vi "主.vi"() -> ()   [LabVIEW 2018]
uses:
  <vilib>/addons/database/Connection.llb/DB Tools Open Connec (String).vi
  <vilib>/addons/database/NI_Database_API.lvlib
  <vilib>/addons/database/Auxilliary.llb/DB Tools DataTypes.ctl
  <vilib>/addons/database/Auxilliary.llb/DB Tools Column Info.ctl
panel:
  out "密码":string[](array[string])
  out "账户":string[](array[string])
  in  "登录":bool
  in  "退出":bool
  in  "密码":string
  in  "用户":string
  in  "数据库路径":path
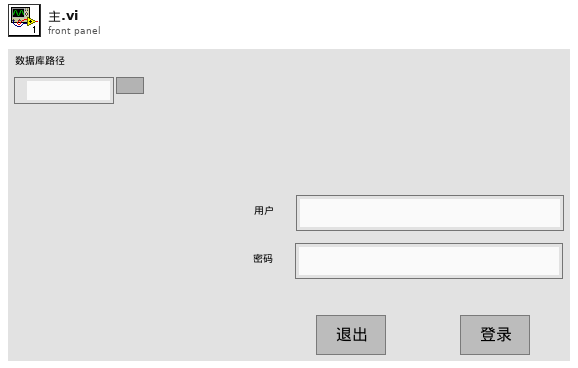
[diagram p1: front panel]
types:
  T1 = typedef "NI_Database_API.lvlib/DB Tools Column Info.ctl" = cluster{"column name":string, "data type":T2, "size":i32, "allow null?":bool}
  T2 = typedef "NI_Database_API.lvlib/DB Tools DataTypes.ctl" = enum16{"String", "Long (I32)", "Single (SGL)", "Double (DBL)", "Date/Time", "Binary"}
  T3 = typedef "NI_Database_API.lvlib/Conn ObjectReference.ctl" = refnum<k1>
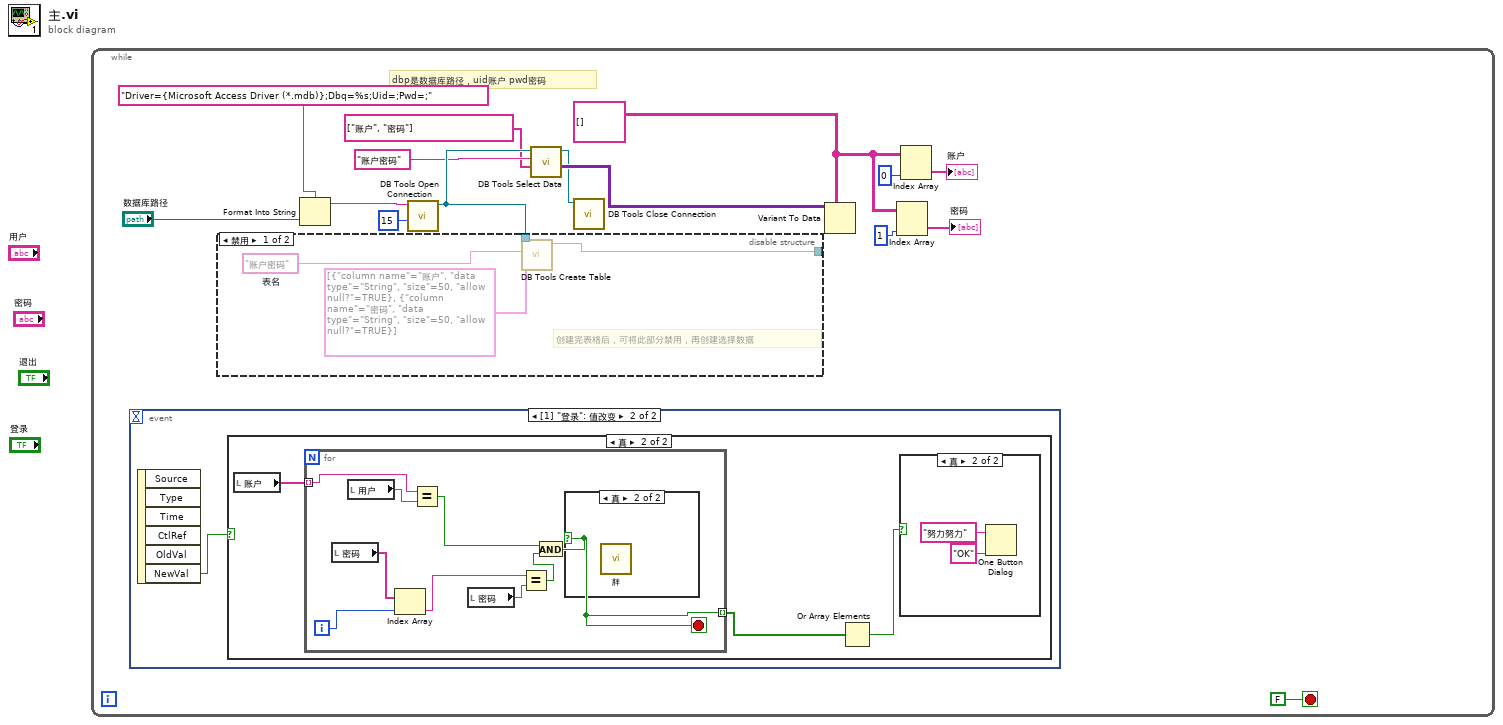
[diagram p0: block diagram]
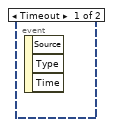
[diagram p3: hidden frame]
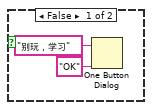
[diagram p6: hidden frame]
diagram:
  n1 = while {
    stop <- FALSE stop-if-true
    w7 = string[][] []
    # "dbp是数据库路径，uid账户 pwd密码"
    n2 = event shown="[1] \"登录\": 值改变" {
      selector: _ -> [_ _]
      dyn-events: _ -> [_ _]
      timeout: _ -> [_ _]
      event Timeout {
        n3 = event-data() -> ()  [unwired: 1 in, 3 out]
      }
      event "登录": Value Change {
        n4 = event-data() -> ("NewVal"=w20:bool)  [unwired: 1 in, 5 out]
        n5 = case shown="真" w20 {
          frame False {
          }
          frame True {
            n6 = local read "账户"() -> (w23:string[])
            n7 = for {
              tunnel: w23 -> [w34] mode=indexing
              tunnel: [w26] -> w21 mode=indexing
              i -> [w32]
              stop <- w26 stop-if-true
              n8 = local read "密码"() -> (w31:string[])
              n9 = local read "用户"() -> (w33:string)
              n10 = Index Array(array=w31, index=w32) -> (element=w30:string)
              n11 = Equal?(x=w34, y=w33) -> (x = y?=w28:bool)
              n12 = local read "密码"() -> (w29:string)
              n13 = Equal?(x=w30, y=w29) -> (x = y?=w27:bool)
              n14 = And(x=w28, y=w27) -> (x .and. y?=w26:bool)
              n15 = case shown="真" w26 {
                frame False {
                  n16 = One Button Dialog(message="别玩，学习" ("消息"), button name ("OK")="OK" ("按钮名称（“确定”）")) -> ()  [unwired: 1 out]
                }
                frame True {
                  n17 = call "胖.vi"() -> ()  [unwired: 12 in]
                }
              }
            }
            n18 = Or Array Elements(Boolean array=w21) -> (logical OR=w22:bool)
            n19 = case shown="真" w22 {
              frame False {
              }
              frame True {
                n20 = One Button Dialog(message="努力努力" ("消息"), button name ("OK")="OK" ("按钮名称（“确定”）")) -> ()  [unwired: 1 out]
              }
            }
          }
        }
      }
    }
    n21 = Format Into String(format string="Driver={Microsoft Access Driver (*.mdb)};Dbq=%s;Uid=;Pwd=;", "数据库路径") -> (resulting string=w13:string)  [unwired: 2 in, 1 out]
    n22 = call-poly <vilib>:"DB Tools Open Connection.vi"("connection timeout (15)"=15, "connection information"=w13) -> ("connection reference"=w11:T3)  [unwired: 6 in, 1 out]
    n23 = disable-structure shown="禁用" {
      disable-tunnel: [w19 _] -> _
      disable-tunnel: w11 -> [w16 _]
      frame Disabled {
        w18 = "账户密码"  # 表名
        # "创建完表格后，可将此部分禁用，再创建选择数据"
        n24 = call <vilib>:"DB Tools Create Table.vi"("column information"=T1[] [{"column name"="账户", "data type"=enum."String", "size"=50, "allow null?"=TRUE}, {"column name"="密码", "data type"=enum."String", "size"=50, "allow null?"=TRUE}], "table"=w18, "connection reference"=w16) -> ("connection reference out"=w19:T3)  [unwired: 5 in, 1 out]
      }
      frame Enabled {
      }
    }
    n25 = call <vilib>:"DB Tools Select Data.vi"("columns"=string[] ["账户", "密码"], "table"="账户密码", "connection reference"=w11) -> ("data"=w8:variant[][], "connection reference out"=w1:T3)  [unwired: 3 in, 1 out]
    n26 = call <vilib>:"DB Tools Close Connection.vi"("connection reference"=w1) -> ()  [unwired: 6 in, 1 out]
    n27 = Variant To Data(type=w7, Variant=w8) -> ()  [unwired: 1 in, 2 out]
    n28 = Index Array(array=w7, index (col)=1 ("禁用的索引 (列)")) -> (element=→"密码":string[])  [unwired: 1 in]
    n29 = Index Array(array=w7, index (col)=0 ("禁用的索引 (列)")) -> (element=→"账户":string[])  [unwired: 1 in]
  }
